vi "NLcalib.vi"(4 "K5":sgl, 5 "V_offset":sgl, 6 "K4":sgl, 7 "Volt QPD":sgl, 8 "K3":sgl, 9 "K2":sgl, 10 "K1":sgl, 11 "K0":sgl) -> (3 "pixels":sgl)   [LabVIEW 2019]
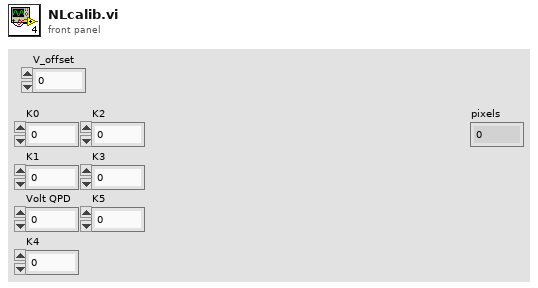
[diagram p1: front panel]
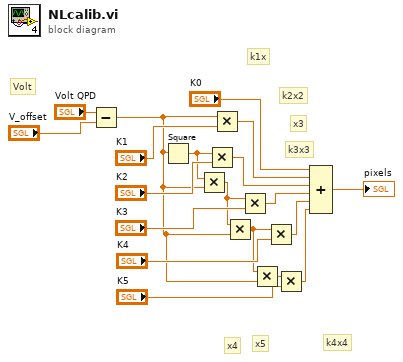
[diagram p0: block diagram]
diagram:
  # "k4x4"
  # "k3x3"
  # "k1x"
  # "x5"
  # "x4"
  # "x3"
  # "k2x2"
  # "Volt"
  n1 = Subtract(x="Volt QPD", y="V_offset") -> (x-y=w3:sgl)
  n2 = Square(x=w3) -> (x^2=w15:sgl)
  n3 = Multiply(x=w15, y=w3) -> (x*y=w8:sgl)
  n4 = Multiply(x=w15, y="K2") -> (x*y=w14:sgl)
  n5 = Multiply(x=w3, y="K1") -> (x*y=w17:sgl)
  n6 = Multiply(x=w8, y=w3) -> (x*y=w1:sgl)
  n7 = Multiply(x=w8, y="K3") -> (x*y=w12:sgl)
  n8 = Multiply(x=w1, y=w3) -> (x*y=w7:sgl)
  n9 = Multiply(x=w1, y="K4") -> (x*y=w9:sgl)
  n10 = Multiply(x=w7, y="K5") -> (x*y=w5:sgl)
  n11 = Compound Arithmetic op=ADD("K0", w17, w14, w12, w9, w5) -> (→"pixels":sgl)
